vi "Generate Polymorphic VI HTML Documentation.vi"(4 "Root Folder Name":string="Toolkit", 5 "Images Destination":path=path "", 6 "Requirement":string="Labstache", 7 "Destination":path=path "", 8 "Error In":errorcluster, 11 "VI":path=path "") -> (0 "Error Out":errorcluster)   [LabVIEW 2018, in "Scripts.lvlib"]
uses:
  Scripts.lvlib
  Toolkit/Data/Array/Array.lvclass
  D:/Users/cfield/Code/Field R&D Services/Mustache/LabVIEW/trunk/src/Toolkit/Data/Datum/Datum.lvclass
  Toolkit/Data/Map/Map.lvclass
  Toolkit/Data/Map/Support/From String.vi
  Toolkit/Data/Map/Support/From Datum.vi
  Toolkit/Data/Map/Support/From Map Array.vi
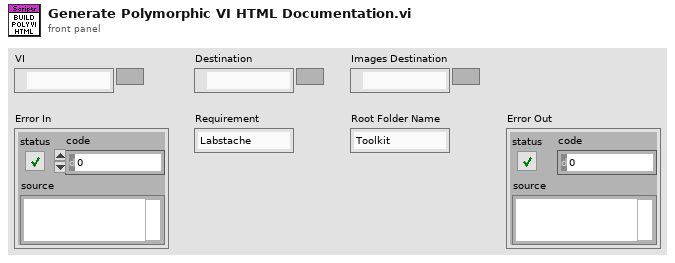
[diagram p1: front panel]
types:
  T1 = cluster{"VIPath":path, "Menu Name":string, "Selector Name":string}[]
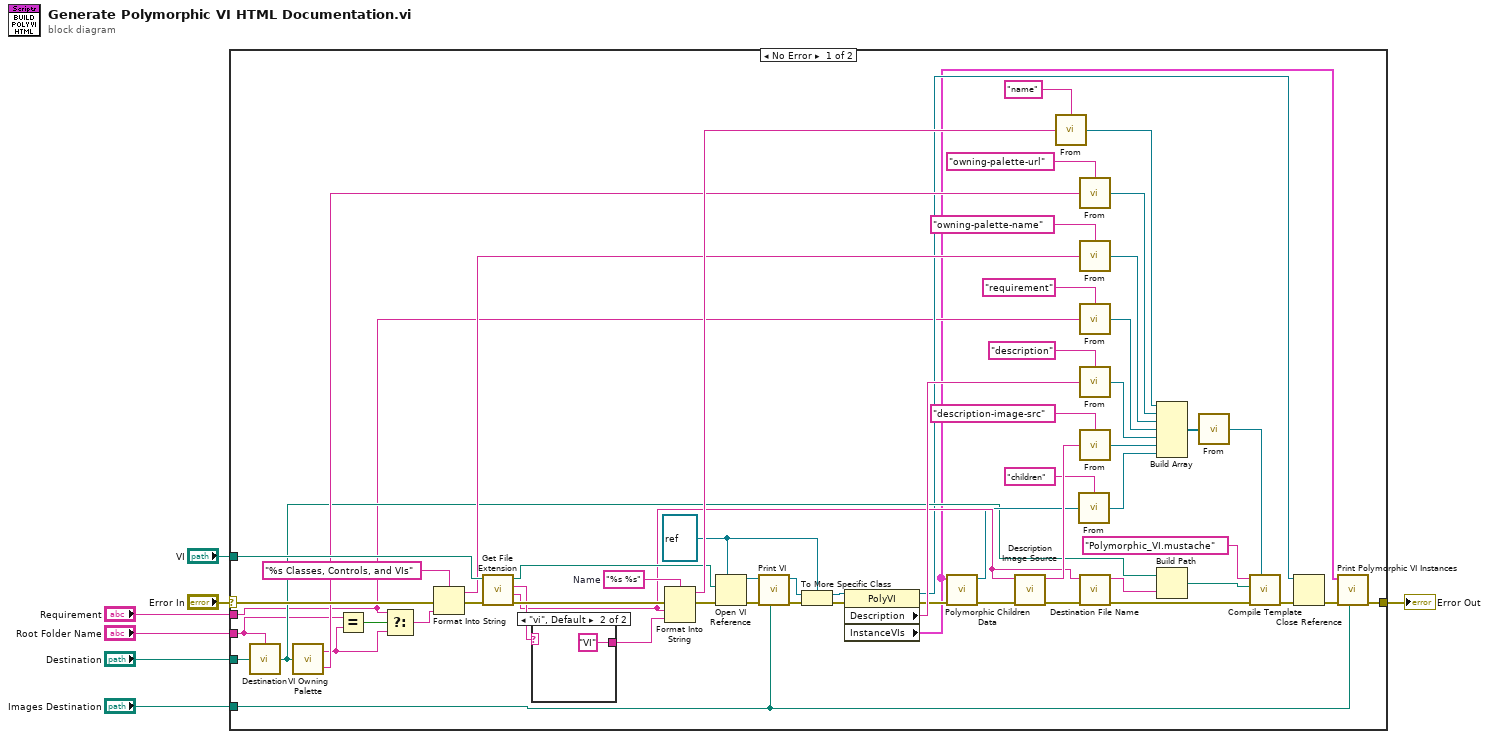
[diagram p0: block diagram]
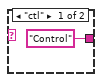
[diagram p2: hidden frame]
diagram:
  n1 = case shown="No Error" "Error In" {
    selector: "Error In" -> [w40 w70]
    tunnel: [w12 w70] -> w7
    tunnel: "VI" -> [w45 _]
    tunnel: "Destination" -> [w14 _]
    tunnel: "Requirement" -> [w13 _]
    tunnel: "Images Destination" -> [w10 _]
    tunnel: "Root Folder Name" -> [w8 _]
    frame No Error {
      w20 = refnum<vi> refnum ("type specifier VI Refnum (for type only)")
      w48 = "%s %s"  # Name
      n2 = call "Destination.vi"("Root Destination In"=w14, "Root Folder Name"=w8) -> ("Root Destination Out"=w28:path)
      n3 = call "VI Owning Palette.vi"("Destination"=w28) -> ("Name"=w26:string, "URL"=w39:string)
      n4 = Equal?(x=w8, y=w26) -> (x = y?=w27:bool)
      n5 = Select(t=w13, s=w27, f=w26) -> (s? t:f=w25:string)
      n6 = Format Into String(format string="%s Classes, Controls, and VIs", error in=w40, w25) -> (resulting string=w41:string, error out=w43:errorcluster)  [unwired: 1 in]
      n7 = call <vilib>:"Get File Extension.vi"("error in (no error)"=w43, "file"=w45) -> ("error out"=w49:errorcluster, "filename without extension"=w37:string, "lowercase file extension"=w47:string, "dup file"=w46:path)  [unwired: 5 in, 1 out]
      n8 = case shown="\"vi\", Default" w47 {
        tunnel: ["Control" "VI"] -> w51
        frame "ctl" {
        }
        frame "vi", Default {
        }
      }
      n9 = Format Into String(format string=w48, error in=w49, w37, w51) -> (resulting string=w53:string, error out=w50:errorcluster)  [unwired: 1 in]
      n10 = Open VI Reference(type specifier VI Refnum (for type only)=w20, vi path=w46, error in (no error)=w50) -> (vi reference=w24:refnum<vi>, error out=w22:errorcluster)  [unwired: 3 in]
      n11 = call "Print VI.vi"("Images Destination"=w10, "Error In"=w22, "VI In"=w24) -> ("Error Out"=w23:errorcluster, "VI Out"=w19:refnum<vi>)  [unwired: 7 in]
      n12 = To More Specific Class(target class=w20, reference=w19, error in=w23) -> (specific class reference=w18:refnum<vi>, error out=w21:errorcluster)
      n13 = property class="PolyVI"(reference=w18, error in=w21) -> (reference out=w16:refnum<vi>, error out=w33:errorcluster, "Description"=w54:string, "InstanceVIs"=w11:T1)
      n14 = call "Polymorphic Children Data.vi"("Error In"=w33, "Instance VIs"=w11) -> ("Error Out"=w32:errorcluster, "Children"=w31:refnum<class "Array.lvclass">)  [unwired: 8 in]
      n15 = call "Description Image Source.vi"("Error In"=w32, "File Stem"=w37) -> ("Error Out"=w38:errorcluster, "Description Image Src"=w56:string)  [unwired: 8 in]
      n16 = call-poly "From.vi"("Value"=w53, "Key"="name") -> ("Map"=w62:refnum<class "Map.lvclass">)
      n17 = call-poly "From.vi"("Value"=w31, "Key"="children") -> ("Map"=w29:refnum<class "Map.lvclass">)
      n18 = call-poly "From.vi"("Value"=w39, "Key"="owning-palette-url") -> ("Map"=w67:refnum<class "Map.lvclass">)
      n19 = call-poly "From.vi"("Value"=w41, "Key"="owning-palette-name") -> ("Map"=w65:refnum<class "Map.lvclass">)
      n20 = call-poly "From.vi"("Value"=w13, "Key"="requirement") -> ("Map"=w63:refnum<class "Map.lvclass">)
      n21 = call-poly "From.vi"("Value"=w54, "Key"="description") -> ("Map"=w61:refnum<class "Map.lvclass">)
      n22 = call-poly "From.vi"("Value"=w56, "Key"="description-image-src") -> ("Map"=w60:refnum<class "Map.lvclass">)
      n23 = call "Destination File Name.vi"("Error In"=w38, "File Stem"=w37) -> ("Error Out"=w59:errorcluster, "Destination File Name"=w44:string)  [unwired: 8 in]
      n24 = Build Array(w62, w67, w65, w63, w61, w60, w29) -> (w36:refnum<class "Map.lvclass">[])
      n25 = Build Path(base path=w28, name or relative path=w44) -> (appended path=w34:path)
      n26 = call-poly "From.vi"("Maps"=w36) -> ("Map"=w35:refnum<class "Map.lvclass">)  [unwired: 1 in]
      n27 = call "Compile Template.vi"("Data"=w35, "Error In"=w59, "Output"=w34, "Template File Name"="Polymorphic_VI.mustache" ("name or relative path")) -> ("Error Out"=w17:errorcluster)  [unwired: 7 in]
      n28 = Close Reference(reference=w16, error in (no error)=w17) -> (error out=w15:errorcluster)
      n29 = call "Print Polymorphic VI Instances.vi"("Images Destination"=w10, "Error In"=w15, "InstanceVIs"=w11) -> ("Error Out"=w12:errorcluster)  [unwired: 8 in]
    }
    frame Error {
    }
  }
  "Error Out" <- w7
